vi "Modify Key.vi"(4 "value":string, 6 "key":string, 8 "error in":errorcluster, 9 "section":string, 10 "key definition":T1, 11 "Configuration File in":T2) -> (0 "error out":errorcluster, 3 "Configuration File out":T2)   [LabVIEW 2012, in "configlib.lvlib"]
uses:
  configlib.lvlib
  Configuration File Definition.ctl
  File Options.ctl
  Key Definition.ctl
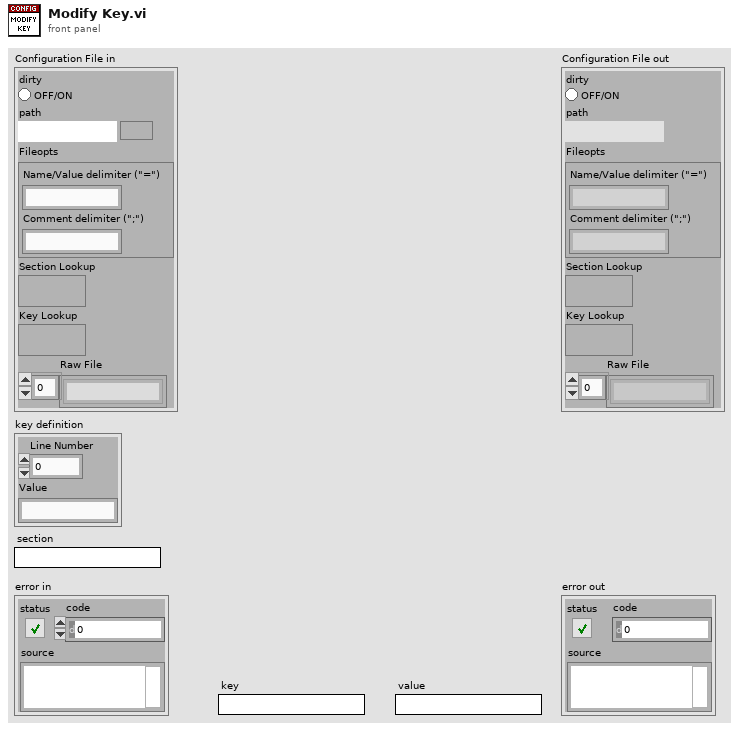
[diagram p1: front panel]
types:
  T1 = typedef "configlib.lvlib/Key Definition.ctl" = cluster{"Line Number":i32, "Value":string}
  T2 = typedef "configlib.lvlib/Configuration File Definition.ctl" = cluster{"dirty":bool, "path":path, "Fileopts":T3, "Section Lookup":variant, "Key Lookup":variant, "Raw File":string[]}
  T3 = typedef "configlib.lvlib/File Options.ctl" = cluster{"Name/Value delimiter (\"=\")":string, "Comment delimiter (\";\")":string}
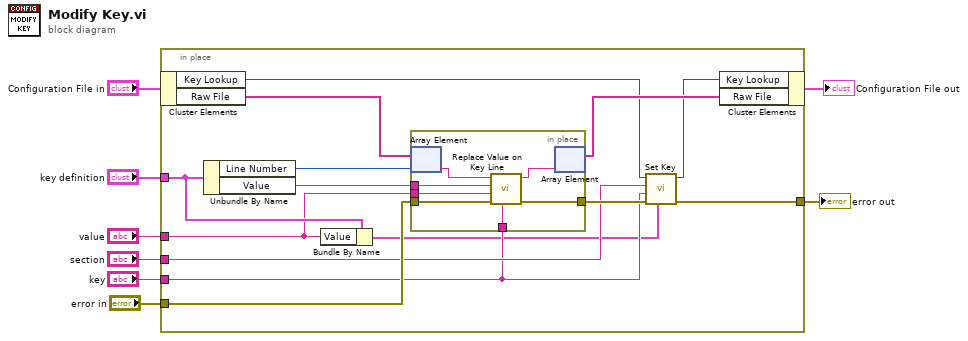
[diagram p0: block diagram]
diagram:
  n1 = in-place {
    in-place-border: "key definition" -> [w21]
    in-place-border: "value" -> [w17]
    in-place-border: "error in" -> [w19]
    in-place-border: "key" -> [w13]
    in-place-border: "section" -> [w14]
    in-place-border: [w9] -> w2
    n2 = in-place-cluster #1("Configuration File in") -> ("Key Lookup"=w11:variant, "Raw File"=w22:string[])
    n3 = Unbundle By Name(w21) -> ("Line Number"=w20:i32, "Value"=w18:string)
    n4 = Bundle By Name(cluster=w21, "Value"=w17) -> (w12:T1)
    n5 = in-place {
      in-place-border: w19 -> [w27]
      in-place-border: [w26] -> w15
      in-place-border: w18 -> [w25]
      in-place-border: w17 -> [w24]
      in-place-border: w13 -> [w23]
      n6 = in-place-array #2(w22, w20) -> (w28:string)
      n7 = call "Replace Value on Key Line.vi"("key"=w23, "error in (no error)"=w27, "new value"=w24, "prev value"=w25, "line in"=w28) -> ("error out"=w26:errorcluster, "line out"=w29:string)  [unwired: 5 in]
      n8 = in-place-array #2(w29) -> (w16:string[])  [unwired: 1 out]
    }
    n9 = call "Set Key.vi"("key definition"=w12, "error in"=w15, "key"=w13, "section"=w14, "key lookup"=w11) -> ("error out"=w9:errorcluster, "key lookup out"=w10:variant)  [unwired: 5 in]
    n10 = in-place-cluster #1("Key Lookup"=w10, "Raw File"=w16) -> (→"Configuration File out":T2)
  }
  "error out" <- w2
